vi "Temperature Monitor (Demo).vi"() -> ()   [LabVIEW 2009]
doc: "Ce VI est un exercice du cours LabVIEW Fondamental 1.\n\nIl est utilisé pour expliquer les boucles While et les graphes déroulants. Ce VI simule une lecture de température toutes les 500 ms et trace les données sur un graphe déroulant."
panel:
  out "Historique de la température":dbl(graph)
  in  "Marche/Arrêt":bool=TRUE
  # "Marche\n\nArrêt"
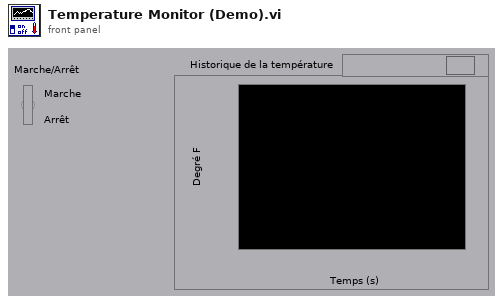
[diagram p1: front panel]
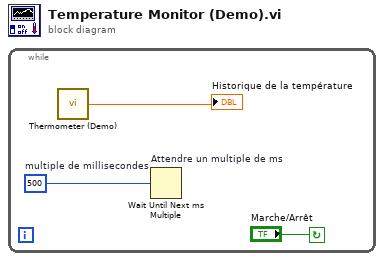
[diagram p0: block diagram]
diagram:
  n1 = while "Boucle While" {
    stop <- "Marche/Arrêt" continue-if-true
    w2 = u32 500  # multiple de millisecondes
    n2 = call "Thermometer (Demo).vi"() -> ("Température"=→"Historique de la température":dbl)  [unwired: 1 in]
    n3 = Wait Until Next ms Multiple "Attendre un multiple de ms"(millisecond multiple=w2) -> ()  [unwired: 1 out]
  }
